vi "writeBrightestToFile.vi"(11 "base path":path) -> ()   [LabVIEW 2012]
uses:
  Cpp Libraries/CatWalkLabviewDLL/labview code/OpenCvGlobals.vi
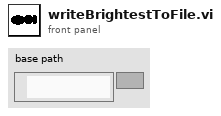
[diagram p1: front panel]
types:
  T1 = enum16{"open", "replace", "create", "open or create", "replace or create", "replace or create with confirmation"}
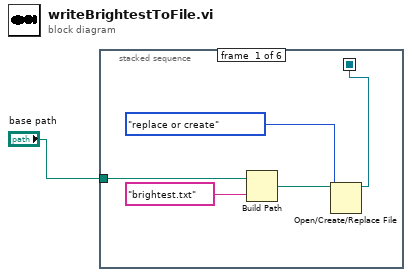
[diagram p0: block diagram]
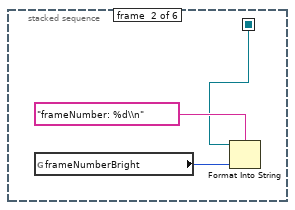
[diagram p2: hidden frame]
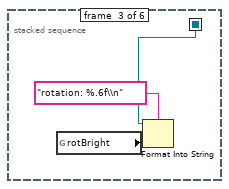
[diagram p3: hidden frame]
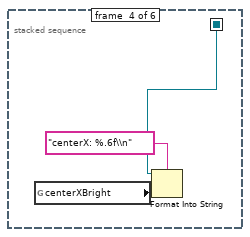
[diagram p4: hidden frame]
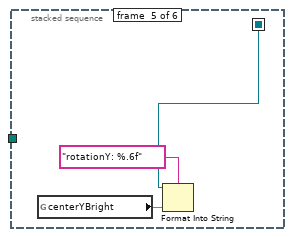
[diagram p5: hidden frame]
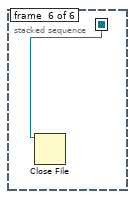
[diagram p6: hidden frame]
diagram:
  n1 = stacked-sequence {
    seq-local: [w4 _ _ _ _ _] -> [_ w7 w12 w13 w16 w19]
    tunnel: "base path" -> [w2 _ _ _ _ _]
    frame #0 {
      n2 = Build Path(base path=w2, name or relative path="brightest.txt") -> (appended path=w5:path)
      n3 = Open/Create/Replace File(file path (use dialog)=w5, operation (0:open)=T1."replace or create") -> (refnum out=w4:refnum<file>)  [unwired: 4 in, 2 out]
    }
    frame #1 {
      n4 = global read "OpenCvGlobals.vi" "frameNumberBright"() -> (w8:i32)
      n5 = Format Into String(format string="frameNumber: %d\\n", initial string=w7, w8) -> ()  [unwired: 1 in, 2 out]
    }
    frame #2 {
      n6 = global read "OpenCvGlobals.vi" "rotBright"() -> (w10:dbl)
      n7 = Format Into String(format string="rotation: %.6f\\n", initial string=w12, w10) -> ()  [unwired: 1 in, 2 out]
    }
    frame #3 {
      n8 = global read "OpenCvGlobals.vi" "centerXBright"() -> (w14:dbl)
      n9 = Format Into String(format string="centerX: %.6f\\n", initial string=w13, w14) -> ()  [unwired: 1 in, 2 out]
    }
    frame #4 {
      n10 = global read "OpenCvGlobals.vi" "centerYBright"() -> (w17:dbl)
      n11 = Format Into String(format string="rotationY: %.6f", initial string=w16, w17) -> ()  [unwired: 1 in, 2 out]
    }
    frame #5 {
      n12 = Close File(refnum=w19) -> ()  [unwired: 1 in, 2 out]
    }
  }
